vi "Rx Streaming (Host).vi"() -> ()   [LabVIEW 2013]
doc: "This template is for the Simple NI-USRP Streaming design, a design that shows the basics of streaming data from an NI 294x/295x device. Refer to the block diagram for more information about how to use this template."
uses:
  <vilib>/userdefined/Silver/nirio_resource_slv.ctl
  SubVIs/Start Trigger.ctl
  <vilib>/Utility/error.llb/DialogType.ctl
  SubVIs/Configure Signal (Level).vi
  SubVIs/Fetch Rx Data (CDB WDT).vi
panel:
  in  "reference frequency source":string(combo)="Internal" caption="Reference Frequency Source"
  in  "antenna":string(combo)="RX1" caption="Active Antenna"
  in  "channel":string(combo)="rx/RF 0" caption="Channel"
  in  "USRP RIO device":T1="RIO0" caption="USRP RIO Device"
  in  "lo frequency":dbl=-1.0 caption="LO Frequency" format="%#.3pHz"
  in  "number of samples is finite":bool=TRUE
  in  "frequency":dbl=2000000000.0 caption="Frequency" format="%#.3pHz"
  in  "sample rate":dbl=10000000.0 caption="Sample Rate" format="%#.3pS/s"
  in  "reference level":dbl caption="Reference Level" format="%#_gdBm"
  in  "start trigger":T2=enum."Immediate" caption="Start Trigger"
  in  "tab control":T3(tab)
  out "Power Spectrum":cluster{"f0":dbl, "df":dbl, "magnitude":dbl[]}(graph)
  out "Power Level":dbl[](graph)
  out "I & Q Data":dbl[][](graph)
  in  "number of samples":u32=8192 caption="Number of Samples"
  in  "stop":bool
  # "Rx Streaming"
  # "This template is for the Simple NI-USRP Streaming design, a design that shows the basics of streaming data from an NI 294x/295x device. See the block diagram for more information on how to use this template."
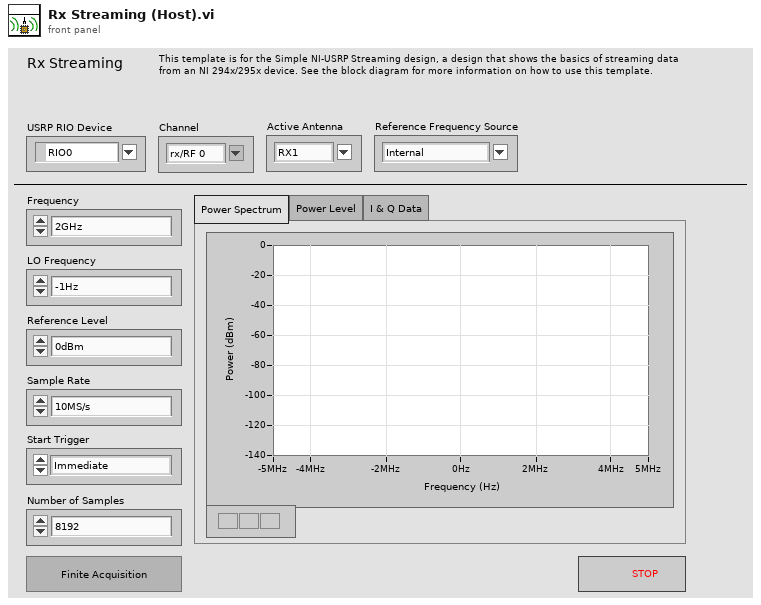
[diagram p1: front panel]
types:
  T1 = typedef "nirio_resource_slv.ctl" = tag
  T2 = typedef "Start Trigger.ctl" = enum8{"Software", "Digital Edge", "Rx Start Trigger", "Tx Start Trigger", "Immediate"}
  T3 = enum32{"Power Spectrum", "Power Level", "I & Q Data"}
  T4 = typedef "DialogType.ctl" = u16
  T5 = typedef "niUsrpRio Config v1 Host.lvlib/niUsrpRio Session.ctl" = cluster{"Global Settings Register Bus":T6, "Radio 0 Settings Register Bus":T6, "Rx NI-USRP session":refnum<k15>, "Tx NI-USRP session":refnum<k15>, "FPGA Interface":refnum<k20>, "RIO Interface Number":u32, "EEPROM Header":T7, "Device Data Header":T8, "EEPROM Characterization Header":T9, "Characterization Data":T10[], "Characterization Data Valid?":bool, "Radio 1 Settings Register Bus":T6, "Radio Settings Bus Semaphore":T12}
  T6 = typedef "niInstr Register Bus v0 Host.lvlib/Register Bus Session.ctl" = refnum<queue>
  T7 = typedef "niUsrpRio Config v1 Host.lvlib/EEPROM Header.ctl" = cluster{"Checksum":u32, "Product Code":u16, "Hardware Current Version":u16, "Hardware Oldest Compatible Version":u16, "EEPROM Map Current Version":u16, "EEPROM Map Oldest Compatible Version":u16, "User Password":string, "Pointer to Factory Header":u32, "Pointer to User Header":u32, "Recommended Interval":u16, "Number of Reserved Bytes":i32, "Number of Daughterboards":u8, "Daughterboard IDs":u16[], "Daughterboard Serial Numbers":string[]}
  T8 = typedef "niUsrpRio Config v1 Host.lvlib/EEPROM Device Data Header.ctl" = cluster{"Checksum":u32, "Number of Channels":u8, "Number of Gain Settings":u16[], "Pointer to Characterization Data":u32[], "Number of Reserved Bytes":i32, "Number of Frequencies":u16[]}
  T9 = typedef "niUsrpRio Config v1 Host.lvlib/EEPROM Characterization Header.ctl" = cluster{"Checksum":u32, "Date":timestamp, "Temperature":sgl, "Misc. Info":string, "Pointer to Device Data Header":u32, "Number of Reserved Bytes":i32}
  T10 = typedef "niUsrpRio Config v1 Host.lvlib/Characterization Data.ctl" = cluster{"Gains[dB]":dbl[], "Frequencies [Hz]":dbl[], "IQ Imbalance Table":T11[], "Measured Gains[dB]":dbl[][]}
  T11 = typedef "niUsrpRio Config v1 Host.lvlib/IQ Imbalance.ctl" = cluster{"Gain Imbalance [linear]":dbl, "Phase Imbalance [radians]":dbl, "Offset":cdb}
  T12 = typedef "Semaphore RefNum" = refnum<k1>
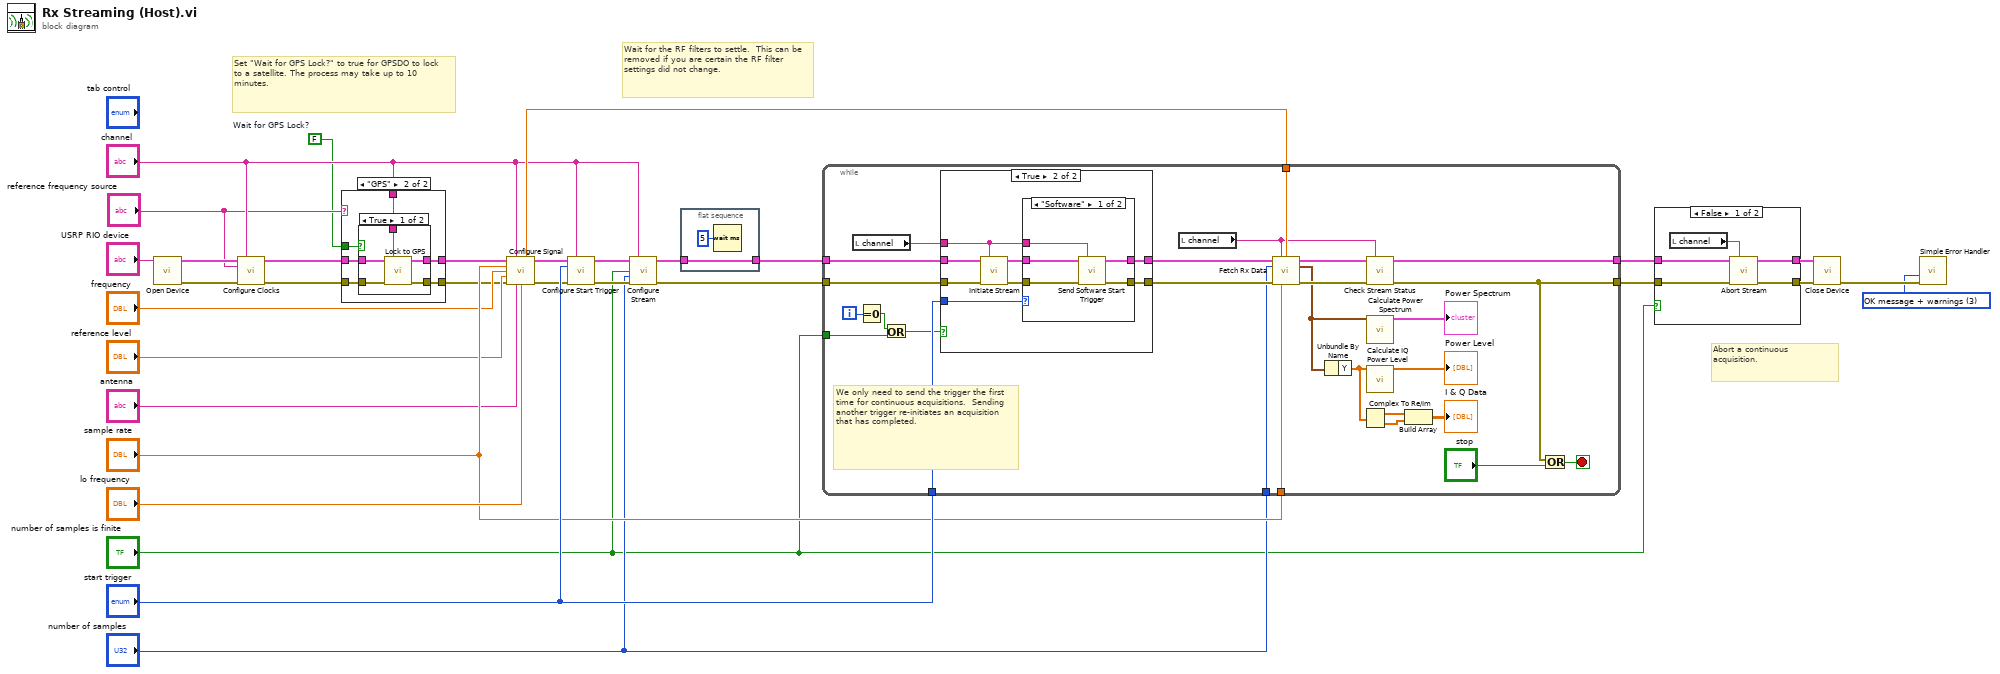
[diagram p0: block diagram]
diagram:
  w1 = FALSE  # Wait for GPS Lock?
  w30 = T4 3 items=["no dialog", "OK message", "continue or stop message", "OK message + warnings", "continue/stop + warnings"] ("type of dialog (OK msg:1)")
  # "Set \"Wait for GPS Lock?\" to true for GPSDO to lock to a satellite. The process may take up to 10 minutes."
  # "Wait for the RF filters to settle.  This can be removed if you are certain the RF filter settings did not change."
  # "Abort a continuous acquisition."
  n1 = call "Open Device.vi"("USRP RIO device"="USRP RIO device") -> ("niUsrpRio Session (out)"=w24:T5, "error out"=w23:errorcluster)  [unwired: 13 in]
  n2 = call "Configure Clocks.vi"("niUsrpRio Session"=w24, "scope"="channel", "Reference Frequency Source"="reference frequency source", "error in"=w23) -> ("niUsrpRio Session (out)"=w7:T5, "error out"=w4:errorcluster)  [unwired: 10 in]
  n3 = case shown="\"GPS\"" "reference frequency source" {
    tunnel: w7 -> [w34 w40]
    tunnel: [w34 w39] -> w6
    tunnel: [w33 w38] -> w5
    tunnel: w4 -> [w33 w37]
    tunnel: "channel" -> [_ w36]
    tunnel: w1 -> [_ w35]
    frame Default {
    }
    frame "GPS" {
      n4 = case shown="True" w35 {
        tunnel: w40 -> [w42 w47]
        tunnel: [w45 w47] -> w39
        tunnel: [w44 w46] -> w38
        tunnel: w37 -> [w41 w46]
        tunnel: w36 -> [w43 _]
        frame True {
          n5 = call "Lock to GPS.vi"("niUsrpRio Session"=w42, "scope"=w43, "error in"=w41) -> ("niUsrpRio Session (out)"=w45:T5, "error out"=w44:errorcluster)  [unwired: 11 in]
        }
        frame False {
        }
      }
    }
  }
  n6 = call-poly "Configure Signal.vi"("niUsrpRio Session"=w6, "scope"="channel", "sample rate [S/s]"="sample rate", "frequency [Hz]"="frequency", "level [dBm]"="reference level", "error in"=w5, "Active Antenna"="antenna", "LO frequency [Hz]"="lo frequency") -> ("coerced vertical range [Vpp]"=w16:dbl, "niUsrpRio Session (out)"=w21:T5, "error out"=w22:errorcluster)  [unwired: 1 in, 4 out]
  n7 = call "Configure Start Trigger.vi"("niUsrpRio Session"=w21, "scope"="channel", "start trigger"="start trigger", "error in"=w22) -> ("niUsrpRio Session (out)"=w20:T5, "error out"=w25:errorcluster)  [unwired: 10 in]
  n8 = call "Configure Stream.vi"("niUsrpRio Session"=w20, "scope"="channel", "number of samples is finite"="number of samples is finite", "number of samples"="number of samples", "error in"=w25) -> ("niUsrpRio Session (out)"=w29:T5, "error out"=w32:errorcluster)  [unwired: 9 in]
  n9 = flat-sequence {
    tunnel: w29 -> [w48]
    tunnel: [w48] -> w28
    frame #0 {
      # "Wait for the RF filters to settle.  This can be removed if you are certain the RF filter settings did not change."
      n10 = Wait (ms)(milliseconds to wait=u32 5) -> ()  [unwired: 1 out]
    }
  }
  n11 = while {
    tunnel: w28 -> [w66]
    tunnel: [w74] -> w14
    tunnel: w16 -> [w58]
    tunnel: "sample rate" -> [w57]
    tunnel: "number of samples" -> [w56]
    tunnel: "start trigger" -> [w69]
    tunnel: w32 -> [w68]
    tunnel: [w73] -> w13
    tunnel: "number of samples is finite" -> [w53]
    i -> [w54]
    stop <- w76 stop-if-true
    # "We only need to send the trigger the first time for continuous acquisitions.  Sending another trigger re-initiates an acquisition that has completed."
    # "Acquire and Fetch a waveform"
    n12 = local read "channel"() -> (w51:string)
    n13 = Equal To 0?(x=w54) -> (x = 0?=w55:bool)
    n14 = Or(x=w55, y=w53) -> (x .or. y?=w52:bool)
    n15 = case shown="True" w52 {
      tunnel: w69 -> [_ w79]
      tunnel: w68 -> [w77 w82]
      tunnel: [w77 w86] -> w67
      tunnel: w66 -> [w78 w84]
      tunnel: [w78 w85] -> w65
      tunnel: w51 -> [_ w80]
      frame False {
      }
      frame True {
        n16 = call "Initiate Stream.vi"("niUsrpRio Session"=w84, "scope"=w80, "error in"=w82) -> ("niUsrpRio Session (out)"=w83:T5, "error out"=w81:errorcluster)  [unwired: 11 in]
        n17 = case shown="\"Software\"" w79 {
          tunnel: w81 -> [w91 w93]
          tunnel: w83 -> [w89 w92]
          tunnel: [w90 w93] -> w86
          tunnel: [w88 w92] -> w85
          tunnel: w80 -> [w87 _]
          frame "Software" {
            # "Send the software trigger to the master device only.  The master will also trigger all slave devices."
            n18 = call "Send Software Start Trigger.vi"("niUsrpRio Session"=w89, "scope"=w87, "error in"=w91) -> ("niUsrpRio Session (out)"=w88:T5, "error out"=w90:errorcluster)  [unwired: 11 in]
          }
          frame Default {
          }
        }
      }
    }
    n19 = local read "channel"() -> (w50:string)
    n20 = call-poly "Fetch Rx Data.vi"("niUsrpRio Session"=w65, "scope"=w50, "vertical range [Vpp]"=w58, "number of samples"=w56, "error in"=w67, "sample rate"=w57) -> ("niUsrpRio Session (out)"=w59:T5, "Waveform (CDB WDT)"=w62:waveform(cdb), "error out"=w64:errorcluster)  [unwired: 7 in]
    n21 = Unbundle By Name(w62) -> ("Y"=w63:cdb[])
    n22 = Complex To Re/Im(x + iy=w63) -> (x=w61:dbl[], y=w60:dbl[])
    n23 = call "Check Stream Status.vi"("niUsrpRio Session"=w59, "scope"=w50, "error in"=w64) -> ("niUsrpRio Session (out)"=w74:T5, "error out"=w73:errorcluster)  [unwired: 10 in, 1 out]
    n24 = call "Calculate Power Spectrum.vi"("IQ Waveform"=w62) -> ("power spectrum (dBm)"=→"Power Spectrum":cluster{"f0":dbl, "df":dbl, "magnitude":dbl[]})  [unwired: 14 in]
    n25 = call "Calculate IQ Power Level.vi"("IQ data"=w63) -> ("power level (dBm)"=→"Power Level":dbl[])  [unwired: 14 in]
    n26 = Build Array(w61, w60) -> (→"I & Q Data":dbl[][])
    n27 = Or(x=w73, y="stop") -> (x .or. y?=w76:bool)
  }
  n28 = case shown="False" "number of samples is finite" {
    tunnel: w14 -> [w98 w100]
    tunnel: w13 -> [w97 w99]
    tunnel: [w96 w100] -> w12
    tunnel: [w95 w99] -> w11
    frame False {
      n29 = local read "channel"() -> (w94:string)
      n30 = call "Abort Stream.vi"("niUsrpRio Session"=w98, "scope"=w94, "error in"=w97) -> ("niUsrpRio Session (out)"=w96:T5, "error out"=w95:errorcluster)  [unwired: 11 in]
    }
    frame True {
    }
  }
  n31 = call "Close Device.vi"("niUsrpRio Session"=w12, "error in"=w11) -> ("error out"=w31:errorcluster)  [unwired: 13 in]
  n32 = call <vilib>:"Simple Error Handler.vi"("type of dialog (OK msg:1)"=w30, "error in (no error)"=w31) -> ()  [unwired: 3 in, 5 out]
